vi "waveanim.vi"   [LabVIEW 2012]
uses:
  <vilib>/addons/internet/NI_InternetTK_Core_VIs.lvlib
panel:
  # "params:\nfreq1 (18.0)\nfreq2 (20.0)\nstepsize(Max(freq2-freq1)/10)\nloop (T)"
types:
  T1 = typedef "CGI Connection Info.ctl" = cluster{"name":string, "type":T2, "session":T3}
  T2 = typedef "CGI Request Type.ctl" = enum16{"cgi", ".spool first", ".spool", ".spool last"}
  T3 = typedef "HTTP Session.ctl" = refnum<k1>
  T4 = typedef "NI_FTP.lvlib/Keyed Array.ctl" = cluster{"keys":string[], "values":string[]}
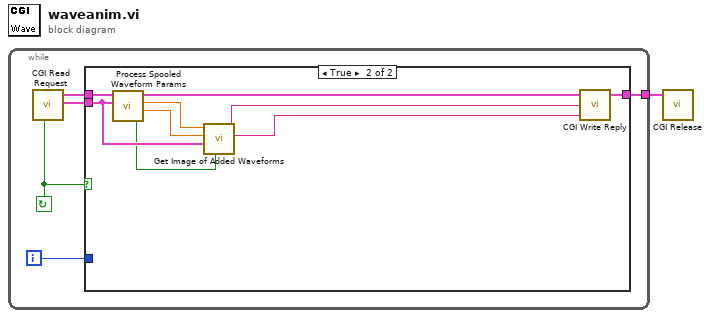
[diagram p0: block diagram]
diagram:
  n1 = while {
    tunnel: [w6] -> w1
    i -> [w2]
    stop <- w4 continue-if-true
    n2 = call <vilib>:"CGI Read Request.vi"() -> ("valid request?"=w4:bool, "cgi connection info"=w5:T1, "env"=w3:T4)  [unwired: 4 in, 1 out]
    n3 = case shown="True" w4 {
      tunnel: [w7 w16] -> w6
      tunnel: w5 -> [w7 w15]
      tunnel: w3 -> [_ w11]
      tunnel: w2 -> [_ _]
      frame False {
      }
      frame True {
        n4 = call "Process Spooled Waveform Params.vi"("env"=w11, "cgi connection info"=w15) -> ("stopping spool"=w8:bool, "cycles 2"=w12:dbl, "cycles 1"=w13:dbl, "cgi connection info out"=w14:T1)  [unwired: 2 in]
        n5 = call "Get Image of Added Waveforms.vi"("close if closed (T)"=w8, "env"=w11, "Cycles 2"=w12, "Cycles 1"=w13) -> ("content"=w9:string, "content header"=w10:string)  [unwired: 5 in, 1 out]
        n6 = call <vilib>:"CGI Write Reply.vi"("content"=w9, "header"=w10, "cgi connection info"=w14) -> ("cgi connection info out"=w16:T1)  [unwired: 2 in]
      }
    }
  }
  n7 = call <vilib>:"CGI Release.vi"("cgi connection info"=w1) -> ()  [unwired: 5 in]
